vi "EventsFGV.vi"(8 "error in":errorcluster, 11 "Command":enum16{"get", "init"}(ring)) -> (0 "error out":errorcluster, 3 "New Event":T1)   [LabVIEW 2013]
uses:
  EventTypDef.ctl
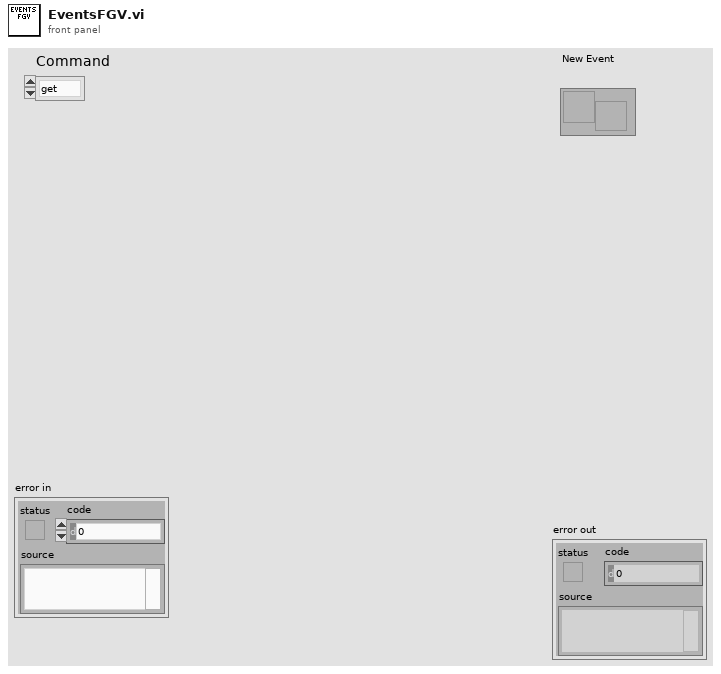
[diagram p1: front panel]
types:
  T1 = typedef "EventTypDef.ctl" = refnum<user-event>
  T2 = cluster{"EventEnum":enum16{"new data", "connection status update"}}
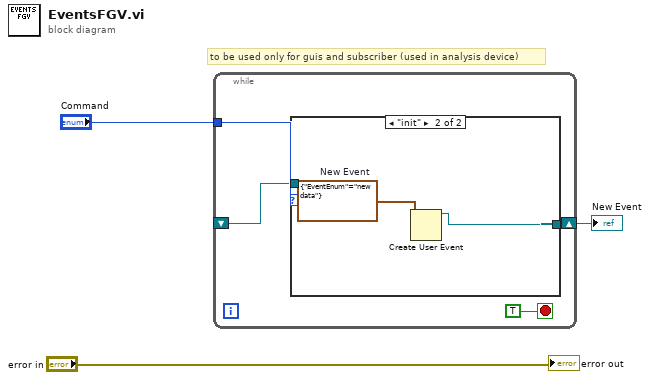
[diagram p0: block diagram]
diagram:
  # "to be used only for guis and subscriber (used in analysis device)"
  n1 = while {
    tunnel: "Command" -> [w6]
    shift-right: [w5] -> w2
    shift-left: _ -> [w4]
    stop <- TRUE stop-if-true
    n2 = case shown="\"init\"" w6 {
      tunnel: [w8 w9] -> w5
      tunnel: w4 -> [w8 _]
      frame "get", Default {
      }
      frame "init" {
        w10 = T2 {"EventEnum"=enum."new data"}  # New Event
        n3 = Create User Event(user event datatype=w10) -> (user event=w9:refnum<user-event>)  [unwired: 1 in, 1 out]
      }
    }
  }
  "New Event" <- w2
  "error out" <- "error in"
